vi "Get Properties.vi"(8 "error in (no error)":errorcluster, 11 "Device Reference In":T1 format="%.0x") -> (0 "error out":errorcluster, 1 "Enable OVP":bool, 2 "ID Query?":bool, 3 "Device Reference Out":T1 format="%.0x", 4 "Voltage Limit":dbl, 5 "Update Rate":u16, 6 "VISA Resource Name":string)   [LabVIEW 2009, in "Agilent 364xA (GPIB,Serial) Custom Device.lvlib"]
uses:
  Agilent 364xA (GPIB,Serial) Custom Device.lvlib
  <vilib>/NI VeriStand/Custom Device API/Custom Device Item Ref.ctl
  <vilib>/NI VeriStand/Custom Device API/Get Item Property (Boolean).vi
  <vilib>/NI VeriStand/Custom Device API/Get Item Property (U16).vi
  <vilib>/NI VeriStand/Custom Device API/Get Item Property (Double).vi
  <vilib>/NI VeriStand/Custom Device API/Get Item Property (String).vi
  Global Strings.vi
  <vilib>/NI VeriStand/Custom Device API/Custom Device API.lvlib
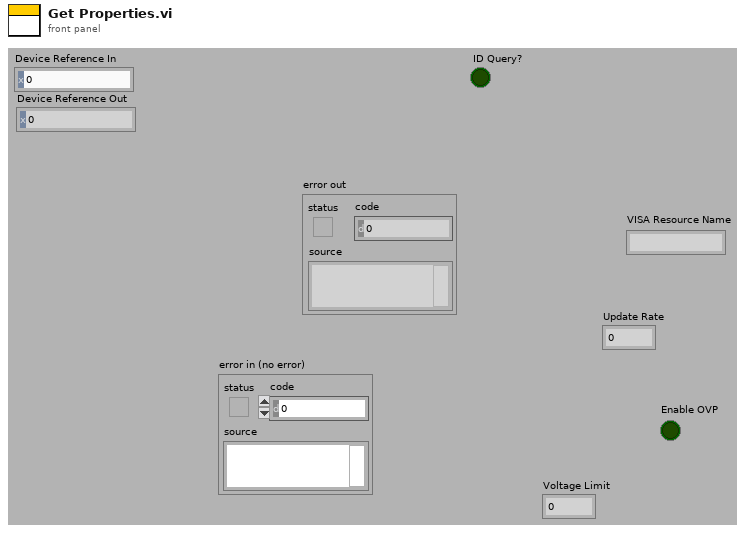
[diagram p1: front panel]
types:
  T1 = typedef "Custom Device API.lvlib/Custom Device Item Ref.ctl" = u64
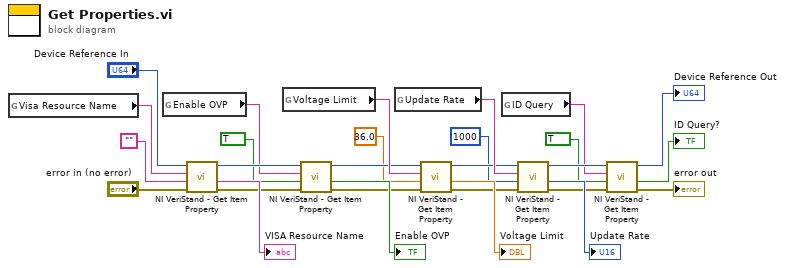
[diagram p0: block diagram]
diagram:
  n1 = global read "Global Strings.vi" "Visa Resource Name"() -> (w25:string)
  n2 = global read "Global Strings.vi" "Enable OVP"() -> (w21:string)
  n3 = call-poly <vilib>:"NI VeriStand - Get Item Property.vi"("error in (no error)"="error in (no error)", "Default Value"="", "Property Name"=w25, "Item Ref in"="Device Reference In") -> ("error out"=w23:errorcluster, "Value"=→"VISA Resource Name":string, "Item Ref out"=w22:T1)  [unwired: 4 in, 1 out]
  n4 = global read "Global Strings.vi" "Voltage Limit"() -> (w19:string)
  n5 = call-poly <vilib>:"NI VeriStand - Get Item Property.vi"("error in (no error)"=w23, "Default Value"=TRUE, "Property Name"=w21, "Item Ref in"=w22) -> ("error out"=w18:errorcluster, "Value"=→"Enable OVP":bool, "Item Ref out"=w17:T1)  [unwired: 4 in, 1 out]
  n6 = global read "Global Strings.vi" "Update Rate"() -> (w14:string)
  n7 = call-poly <vilib>:"NI VeriStand - Get Item Property.vi"("error in (no error)"=w18, "Default Value"=36.0, "Property Name"=w19, "Item Ref in"=w17) -> ("error out"=w15:errorcluster, "Value"=→"Voltage Limit":dbl, "Item Ref out"=w13:T1)  [unwired: 4 in, 1 out]
  n8 = global read "Global Strings.vi" "ID Query"() -> (w9:string)
  n9 = call-poly <vilib>:"NI VeriStand - Get Item Property.vi"("error in (no error)"=w15, "Default Value"=u16 1000, "Property Name"=w14, "Item Ref in"=w13) -> ("error out"=w11:errorcluster, "Value"=→"Update Rate":u16, "Item Ref out"=w10:T1)  [unwired: 4 in, 1 out]
  n10 = call-poly <vilib>:"NI VeriStand - Get Item Property.vi"("error in (no error)"=w11, "Default Value"=TRUE, "Property Name"=w9, "Item Ref in"=w10) -> ("error out"=→"error out":errorcluster, "Value"=→"ID Query?":bool, "Item Ref out"=→"Device Reference Out":T1)  [unwired: 4 in, 1 out]
